vi "Read Cursor Positions.vi"(4 "error in (no error)":errorcluster, 6 "Container State":T4, 7 "Display State In":T1={"Graph Visible Items"={"Plot Legend"=FALSE, "Scale Legend"=FALSE, "Graph Palette"=FALSE, "Cursor Legend"=FALSE, "X Scrollbar"=FALSE}, "View Table"=FALSE, "Table Visible Items"={"Vertical Scrollbar"=FALSE, "Horizontal Scrollbar"=FALSE, "Row Headers"=FALSE, "Column Headers"=FALSE, "Vertical Lines"=FALSE, "Horizontal Lines"=FALSE}, "Header Font"={"Font Name"="", "Size"=0, "Bold"=FALSE, "Italic"=FALSE, "Underline"=FALSE, "Strikeout"=FALSE, "Color"=0}, "Cell Font"={"Font Name"="", "Size"=0, "Bold"=FALSE, "Italic"=FALSE, "Underline"=FALSE, "Strikeout"=FALSE, "Color"=0}, "Description and Tip..."={"Description"="", "Tip"=""}, "Moveable Splitter Position"=0, "Measurement Cursor Configuration"={"relative to t0"={"enable relative time"=FALSE, "Relative times (DT)"=[], "color"=0}, "range"={"enable range"=FALSE, "T1"=0.0, "T2"=0.0, "Fixed interval (T2-T1)"=0.0, "T1 color"=0, "T2 color"=0, "enable shading"=FALSE}, "periodic"={"enable periodic"=FALSE, "First event (E1)"=0.0, "Number events (Ei)"=0, "Event spacing (s)"=0.0, "First color"=0, "Events color"=0}, "absolute timestamp"={"enable absolute"=FALSE, "Timestamps (TS)"=[], "color"=0}}, "X Increment"=0.0, "X Scale"={"Label Visible"=FALSE, "Label Text"="", "Time Mode"=enum."Relative", "Format String"=""}, "Y Scale"={"Label Visible"=FALSE, "Label Text"="", "Scaling"=enum."Engineering Units", "Format String"=""}, "Colors"={"background"=16777215, "major grid"=8355711, "minor grid"=12632256, "font"=0}, "Cursors"={"List"=[], "Tags"=[]}, "Plots"=[], "Plot Color Wheel"=[3381759, 32768, 982784, 4375295, 13827953, 13457919, 16757522, 4343295, 16728758, 12095254], "registered user events"=variant}) -> (0 "error out":errorcluster, 2 "Value":T5, 3 "Display State Out":T1={"Graph Visible Items"={"Plot Legend"=FALSE, "Scale Legend"=FALSE, "Graph Palette"=FALSE, "Cursor Legend"=FALSE, "X Scrollbar"=FALSE}, "View Table"=FALSE, "Table Visible Items"={"Vertical Scrollbar"=FALSE, "Horizontal Scrollbar"=FALSE, "Row Headers"=FALSE, "Column Headers"=FALSE, "Vertical Lines"=FALSE, "Horizontal Lines"=FALSE}, "Header Font"={"Font Name"="", "Size"=0, "Bold"=FALSE, "Italic"=FALSE, "Underline"=FALSE, "Strikeout"=FALSE, "Color"=0}, "Cell Font"={"Font Name"="", "Size"=0, "Bold"=FALSE, "Italic"=FALSE, "Underline"=FALSE, "Strikeout"=FALSE, "Color"=0}, "Description and Tip..."={"Description"="", "Tip"=""}, "Moveable Splitter Position"=0, "Measurement Cursor Configuration"={"relative to t0"={"enable relative time"=FALSE, "Relative times (DT)"=[], "color"=0}, "range"={"enable range"=FALSE, "T1"=0.0, "T2"=0.0, "Fixed interval (T2-T1)"=0.0, "T1 color"=0, "T2 color"=0, "enable shading"=FALSE}, "periodic"={"enable periodic"=FALSE, "First event (E1)"=0.0, "Number events (Ei)"=0, "Event spacing (s)"=0.0, "First color"=0, "Events color"=0}, "absolute timestamp"={"enable absolute"=FALSE, "Timestamps (TS)"=[], "color"=0}}, "X Increment"=0.0, "X Scale"={"Label Visible"=FALSE, "Label Text"="", "Time Mode"=enum."Relative", "Format String"=""}, "Y Scale"={"Label Visible"=FALSE, "Label Text"="", "Scaling"=enum."Engineering Units", "Format String"=""}, "Colors"={"background"=16777215, "major grid"=8355711, "minor grid"=12632256, "font"=0}, "Cursors"={"List"=[], "Tags"=[]}, "Plots"=[], "Plot Color Wheel"=[3381759, 32768, 982784, 4375295, 13827953, 13457919, 16757522, 4343295, 16728758, 12095254], "registered user events"=variant})   [LabVIEW 2017, in "Waveforms with Cursors.xctl"]
uses:
  <vilib>/addons/_XControls/Waveforms with Cursors/Waveforms with Cursors.xctl
  <vilib>/_xctls/Container State.ctl
  <vilib>/addons/_XControls/Waveforms with Cursors/Controls/Cursor Positions.ctl
  <vilib>/addons/_XControls/Waveforms with Cursors/Controls/State.ctl
  <vilib>/Utility/miscctls.llb/LVFontTypeDef.ctl
  <vilib>/addons/_XControls/Waveforms with Cursors/Controls/Waveform Cursor Configuration.ctl
  <vilib>/addons/_XControls/Waveforms with Cursors/Controls/Data.ctl
  <vilib>/Waveform/WDTOps.llb/WDT Get XY Value DBL.vi
  <vilib>/addons/_NISVFA/_Shared subVIs/Common/svc_Engineering Units to Unit Label.vi
  <vilib>/addons/_NISVFA/_Shared subVIs/Common/svc_Unit Label to Engineering Units.vi
  <vilib>/_xctls/XControlSupport.lvlib
panel:
  # "Replace the Value Indicator below with an Indicator of desired type.\nDo not remove this Indicator or the others from the connector pane. \nDo not change the connector pane pattern.\nThe Value Indicator should always be the second terminal from top on the output side in the connector pane."
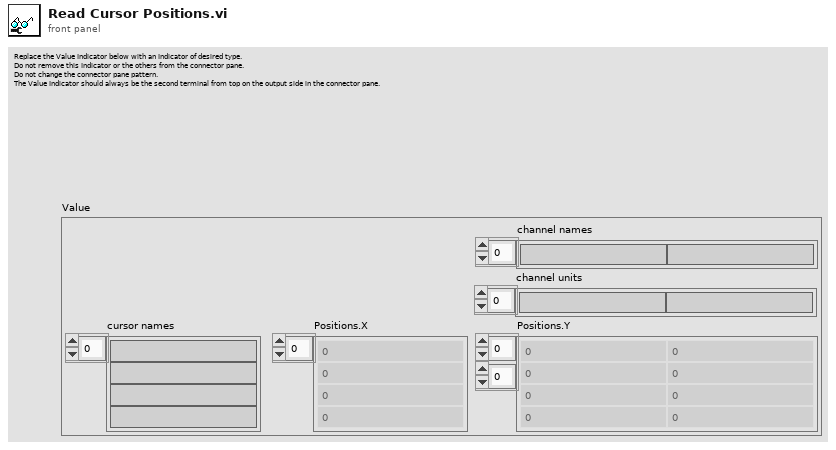
[diagram p1: front panel]
types:
  T1 = typedef "Waveforms with Cursors.xctl/State.ctl" = cluster{"Graph Visible Items":cluster{"Plot Legend":bool, "Scale Legend":bool, "Graph Palette":bool, "Cursor Legend":bool, "X Scrollbar":bool}, "View Table":bool, "Table Visible Items":cluster{"Vertical Scrollbar":bool, "Horizontal Scrollbar":bool, "Row Headers":bool, "Column Headers":bool, "Vertical Lines":bool, "Horizontal Lines":bool}, "Header Font":T2, "Cell Font":T2, "Description and Tip...":cluster{"Description":string, "Tip":string}, "Moveable Splitter Position":i32, "Measurement Cursor Configuration":T3, "X Increment":dbl, "X Scale":cluster{"Label Visible":bool, "Label Text":string, "Time Mode":enum16{"Relative", "Absolute"}, "Format String":string}, "Y Scale":cluster{"Label Visible":bool, "Label Text":string, "Scaling":enum16{"Engineering Units", "Voltage"}, "Format String":string}, "Colors":cluster{"background":u32, "major grid":u32, "minor grid":u32, "font":u32}, "Cursors":cluster{"List":cluster{"Name":string, "Color":u32, "Style":i32, "Point Style":u8, "Name Visible":bool, "Allow Drag":bool, "Cursor Mode":u32, "Plot":i32, "Index":i32, "Position":cluster{"X":dbl, "Y":dbl}, "X Scale":u32, "Y Scale":u32, "Watch Plots":i32[], "Watch All Plots":bool, "Plot Area":i32, "Label Offset":cluster{"X":dbl, "Y":dbl}}[], "Tags":variant[]}, "Plots":cluster{"Name":string, "Line Color":u32, "Line Style":u8, "Line Width":u8, "Fill/Point Color":u32, "Point Style":u8, "Fill To":i16, "Interpolation":u8, "Anti-aliased":bool}[], "Plot Color Wheel":u32[], "registered user events":variant}
  T2 = typedef "LVFontTypeDef.ctl" = cluster{"Font Name":string, "Size":u16, "Bold":bool, "Italic":bool, "Underline":bool, "Strikeout":bool, "Color":u32}
  T3 = typedef "Waveforms with Cursors.xctl/Waveform Cursor Configuration.ctl" = cluster{"relative to t0":cluster{"enable relative time":bool, "Relative times (DT)":dbl[], "color":u32}, "range":cluster{"enable range":bool, "T1":dbl, "T2":dbl, "Fixed interval (T2-T1)":dbl, "T1 color":u32, "T2 color":u32, "enable shading":bool}, "periodic":cluster{"enable periodic":bool, "First event (E1)":dbl, "Number events (Ei)":i32, "Event spacing (s)":dbl, "First color":u32, "Events color":u32}, "absolute timestamp":cluster{"enable absolute":bool, "Timestamps (TS)":timestamp[], "color":u32}}
  T4 = typedef "XControlSupport.lvlib/Container State.ctl" = cluster{"Indicator?":bool, "Run Mode?":bool, " Refnum":refnum<vi>}
  T5 = typedef "Waveforms with Cursors.xctl/Cursor Positions.ctl" = cluster{"cursor names":string[], "channel names":string[], "channel units":string[], "Positions.X":dbl[], "Positions.Y":dbl[][]}
  T6 = typedef "Waveforms with Cursors.xctl/Data.ctl" = waveform(dbl)[]
  T7 = cluster{"Name":string, "Color":u32, "Style":i32, "Point Style":u8, "Name Visible":bool, "Allow Drag":bool, "Cursor Mode":u32, "Plot":i32, "Index":i32, "Position":cluster{"X":dbl, "Y":dbl}, "X Scale":u32, "Y Scale":u32, "Watch Plots":i32[], "Watch All Plots":bool, "Plot Area":i32, "Label Offset":cluster{"X":dbl, "Y":dbl}}[]
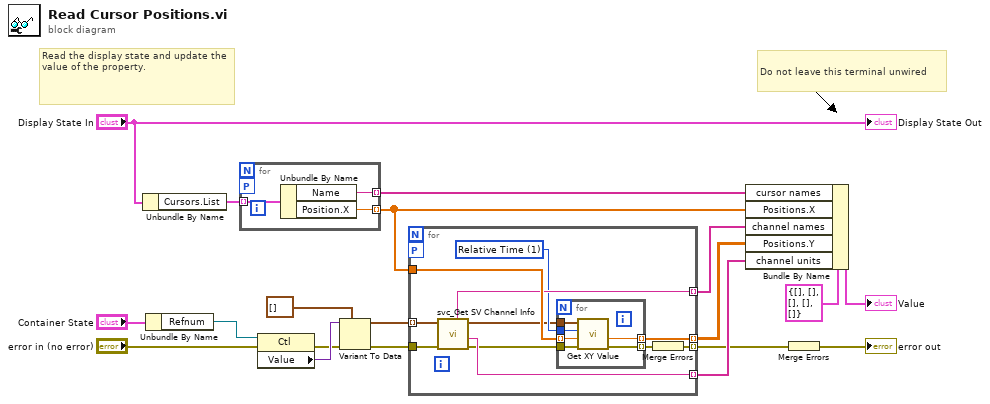
[diagram p0: block diagram]
diagram:
  # "Do not leave this terminal unwired"
  # "Read the display state and update the value of the property."
  n1 = Unbundle By Name("Display State In") -> ("Cursors.List"=w15:T7)
  n2 = Unbundle By Name("Container State") -> ("Refnum"=w18:refnum<vi>)
  n3 = for {
    tunnel: w15 -> [w22] mode=indexing
    tunnel: [w21] -> w14 mode=indexing
    tunnel: [w20] -> w7 mode=indexing
    workers-P: _ -> [_]
    n4 = Unbundle By Name(w22) -> ("Name"=w21:string, "Position.X"=w20:dbl)
  }
  n5 = property class="Ctl"(reference=w18, error in="error in (no error)") -> (error out=w13:errorcluster, "Value"=w17:variant)  [unwired: 1 out]
  n6 = Variant To Data(error in=w13, type=T6 [] ("signals [V]"), Variant=w17) -> (data=w9:T6, error out=w5:errorcluster)
  n7 = for {
    tunnel: [w29] -> w1 mode=indexing
    tunnel: w9 -> [w31] mode=indexing
    tunnel: [w33] -> w8 mode=indexing
    tunnel: w7 -> [w32]
    tunnel: [w30] -> w6 mode=indexing
    workers-P: _ -> [_]
    tunnel: w5 -> [w28]
    tunnel: [w27] -> w4 mode=indexing
    w25 = u16 1 items=["Samples", "Relative Time"] ("Y position format")
    n8 = call <vilib>:"svc_Get SV Channel Info.vi"("error in (no error)"=w28, "scaled signal [EU]"=w31) -> ("error out"=w23:errorcluster, "unit label"=w33:string, "dup scaled signal [EU]"=w24:waveform(dbl), "channel name"=w29:string)  [unwired: 4 in, 2 out]
    n9 = for {
      tunnel: w32 -> [w39] mode=indexing
      tunnel: w24 -> [w38]
      tunnel: [w37] -> w30 mode=indexing
      tunnel: w25 -> [w36]
      tunnel: w23 -> [w35]
      tunnel: [w34] -> w26 mode=indexing
      n10 = call-poly <vilib>:"Get XY Value.vi"("error in (no error)"=w35, "Y position"=w39, "Y position format"=w36, "waveform in"=w38) -> ("error out"=w34:errorcluster, "Y value"=w37:dbl)  [unwired: 3 in, 3 out]
    }
    n11 = Merge Errors(w26) -> (w27:errorcluster)
  }
  n12 = Bundle By Name(cluster=T5 {"cursor names"=[], "channel names"=[], "channel units"=[], "Positions.X"=[], "Positions.Y"=[]} ("Value"), "cursor names"=w14, "Positions.X"=w7, "channel names"=w1, "Positions.Y"=w6, "channel units"=w8) -> (→"Value":T5)
  n13 = Merge Errors(w4) -> (→"error out":errorcluster)
  "Display State Out" <- "Display State In"
